vi "Load.vi"(7 "Renderer":u32, 8 "error in (no error)":errorcluster, 10 "Scale":sgl=1.0, 11 "Path":path) -> (0 "error out":errorcluster, 2 "Pixels":u32[][](array[numeric]), 3 "Texture out":refnum<class "Texture.lvclass">)   [LabVIEW 2021, in "Texture.lvclass"]
uses:
  Texture.lvclass
  Texture.lvclass/Texture.ctl
  LabSDL2/Source/Libraries/SDL2 Utility/SDL2 Utility.lvlib
  LabSDL2/Source/Libraries/LibSDL2 Wrapper/Controls/RGB.ctl
  LabSDL2/Source/Libraries/LibSDL2 Wrapper/LibSDL2.lvlib
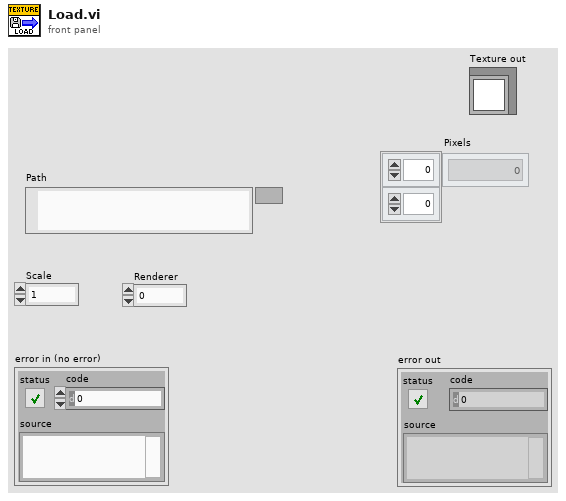
[diagram p1: front panel]
types:
  T1 = typedef "LibSDL2.lvlib/RGB.ctl" = cluster{"R":u8, "G":u8, "B":u8}
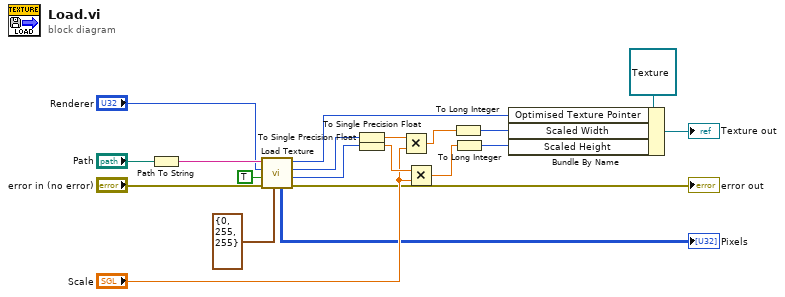
[diagram p0: block diagram]
diagram:
  n1 = Path To String(path="Path") -> (string=w17:string)
  n2 = call "Load Texture.vi"("RGB"=T1 {"R"=0, "G"=255, "B"=255}, "error in"="error in (no error)", "Apply Colour Key (F)"=TRUE, "Renderer Pointer"="Renderer", "File"=w17) -> ("error out"=→"error out":errorcluster, "Height"=w12:i32, "Width"=w13:i32, "Optimised Texture Pointer"=w16:u32, "Pixels"=→"Pixels":u32[][])  [unwired: 2 in]
  n3 = To Single Precision Float(number=w13) -> (single precision float=w11:sgl)
  n4 = To Single Precision Float(number=w12) -> (single precision float=w8:sgl)
  n5 = Multiply(x=w11, y="Scale") -> (x*y=w10:sgl)
  n6 = Multiply(x=w8, y="Scale") -> (x*y=w6:sgl)
  n7 = To Long Integer(number=w10) -> (32bit integer=w9:i32)
  n8 = To Long Integer(number=w6) -> (32bit integer=w5:i32)
  n9 = Bundle By Name(cluster=refnum<class "Texture.lvclass"> refnum ("Texture in"), "Optimised Texture Pointer"=w16, "Scaled Width"=w9, "Scaled Height"=w5) -> (→"Texture out":refnum<class "Texture.lvclass">)
